vi "Branched Log Example.vi"() -> ()   [LabVIEW 2019]
doc: "This example shows logging data from multiple loops. At first, only one sink is active and then when another is added both loops will write to both logs (even though the wire is branched and isn't \"directly\" connected to the wire where the second sink is added.\n\nThis shows the DVR capability and the flexibility for event logs to be added on the fly."
uses:
  Log/Event Level.ctl
  Log/Log.lvclass/Log.ctl
  Layouts/JSONLayout/JSONLayout.lvclass
  C:/Development/Open Source/tsc-event-logger/Layouts/Layout.lvclass
  9e8dcfb1-bbfa-4add-8900-7eeb32d884c9.vi
  6aea5bb5-3dcc-47de-b7f9-df75227292dc.vi
  Log/Read Sinks.vi
  Log Sinks/Sink-Console/Sink-Console.lvclass
  C:/Development/Open Source/tsc-event-logger/Log Sinks/Log Sinks.lvclass
  Log Sinks/Sink-Console/Construct - Input.vi
  Log Sinks/Send Log Packet.vi
  Log/Log.lvclass
  TSC Event Logger.lvlib
panel:
  out "Closed?":bool
  in  "Arguments":string[](array[string])
  in  "Bottom Level":T1=enum."INFO"
  in  "Record Bottom Event":bool
  in  "Bottom Message":string="test"
  in  "Add JSON Console":bool
  out "Second Console":string
  out "First Console":string
  in  "Level":T1=enum."INFO"
  in  "Record Event":bool
  in  "Message":string="test"
  out "Error Out":errorcluster
  # "Run VI: both loops should be able to log to first console. \nThe second console is added with the add button in the top loop. \n-->Will the second console get the bottom loop messages after that?????"
  # "Top-Loop"
  # "Bottom-Loop"
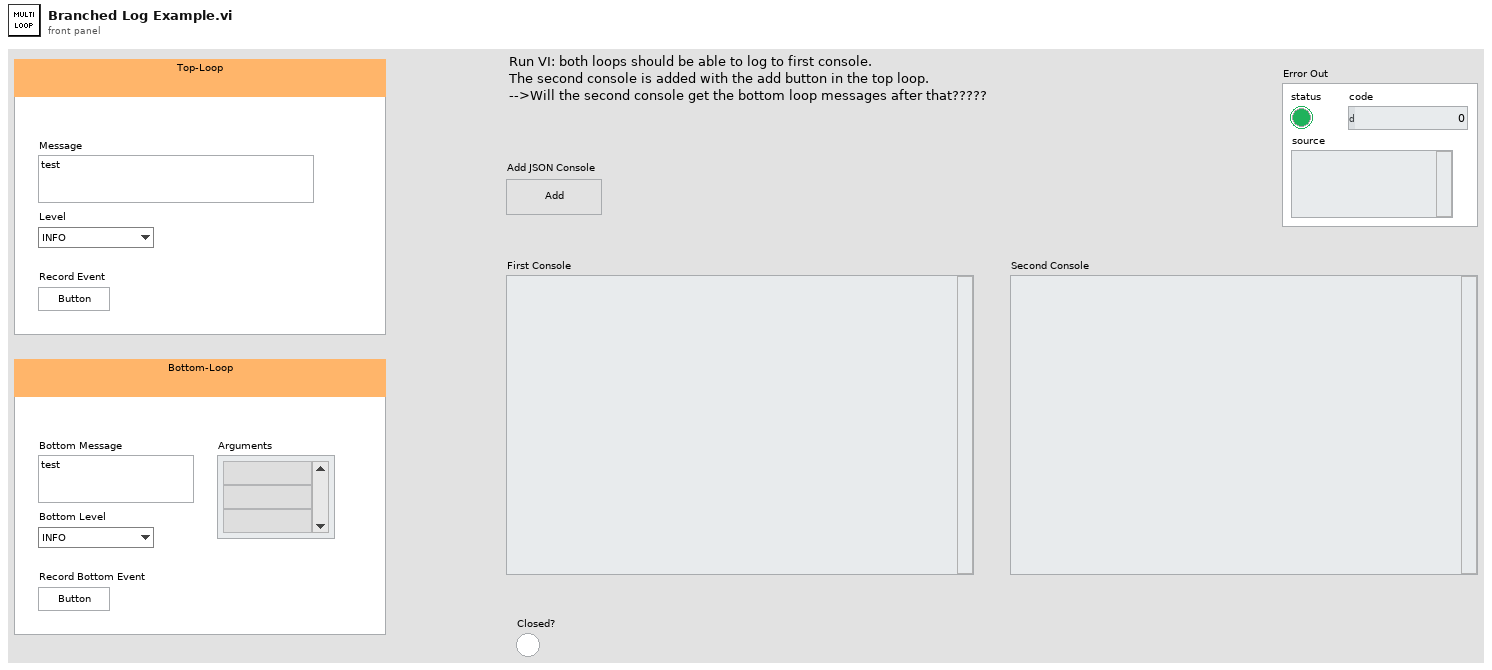
[diagram p1: front panel]
types:
  T1 = typedef "TSC Event Logger.lvlib/Event Level.ctl" = enum16{"OFF", "TRACE", "DEBUG", "INFO", "WARN", "ERROR", "FATAL"}
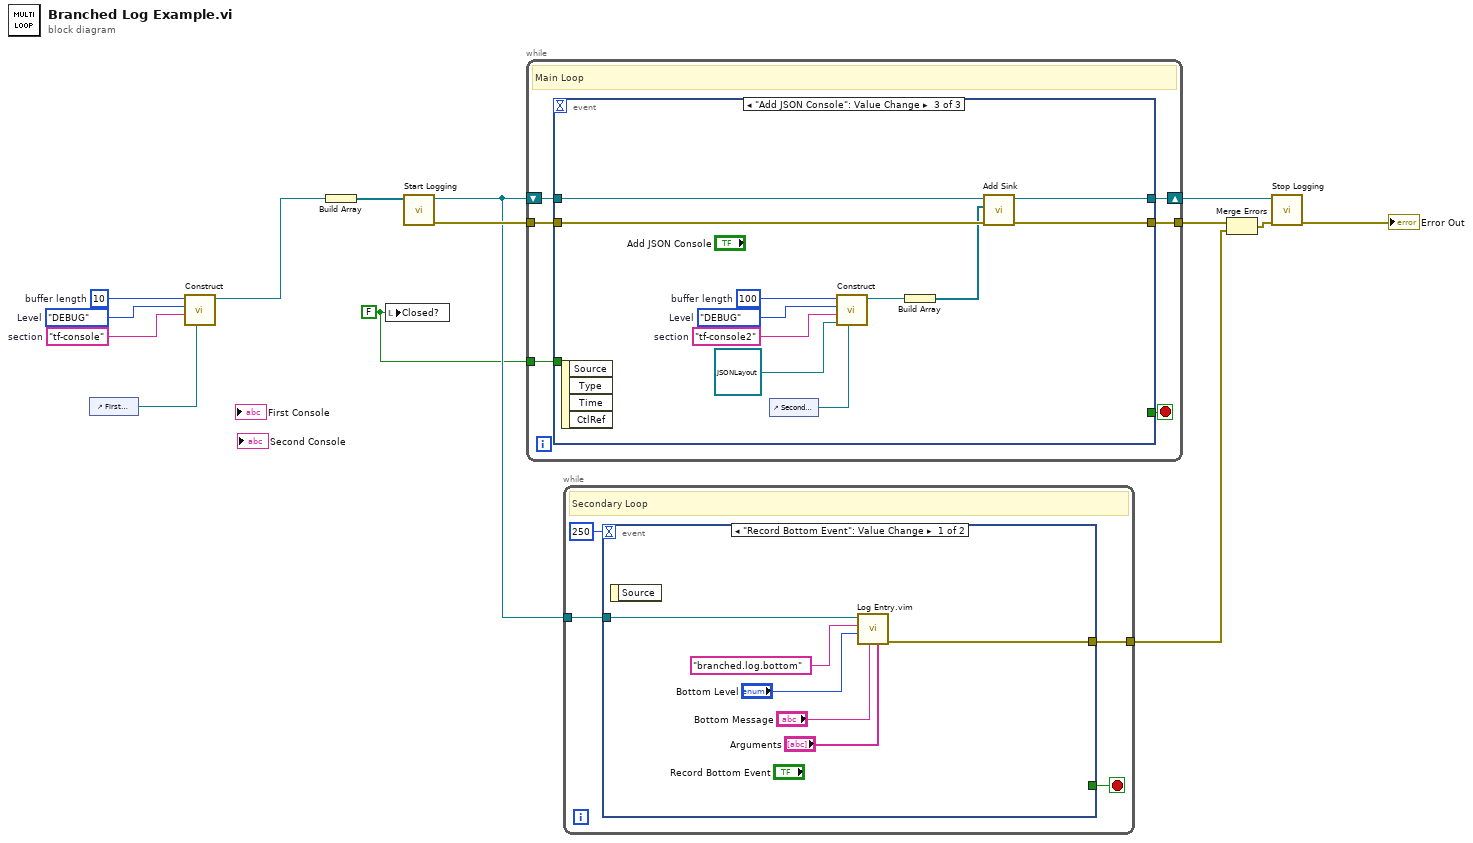
[diagram p0: block diagram]
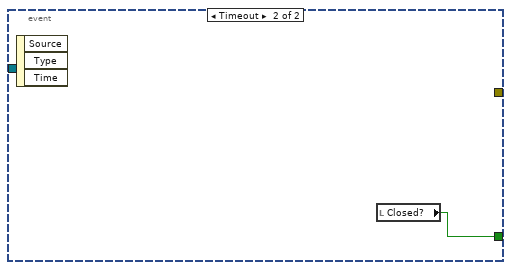
[diagram p2: hidden frame]
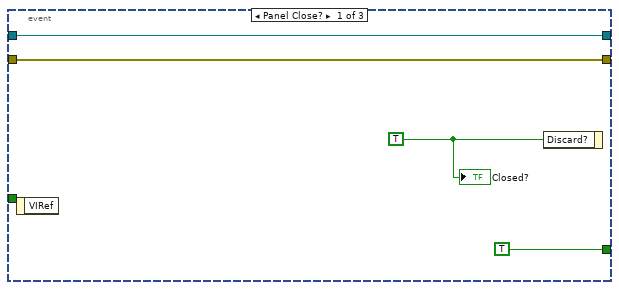
[diagram p3: hidden frame]
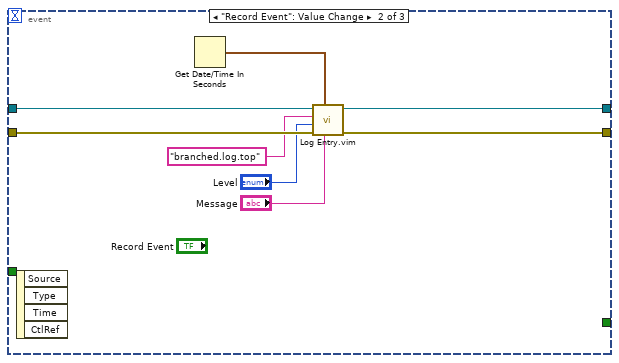
[diagram p4: hidden frame]
diagram:
  w1 = FALSE ("Closed?")
  w5 = 10  # buffer length
  w6 = Event_Level."DEBUG"  # Level
  w7 = "tf-console"  # section
  n1 = control-ref of="First Console"() -> (w8:refnum<vi>)
  n2 = call-poly "Construct.vi"("Console Ref"=w8, "Name"=w7, "Level"=w6, "buffer length"=w5) -> ("Sink-Console"=w9:refnum<class "Sink-Console.lvclass">)  [unwired: 6 in, 1 out]
  n3 = Build Array(w9) -> (w10:refnum<class "Sink-Console.lvclass">[])
  n4 = local write "Closed?"(w1) -> ()
  n5 = call "Start Logging.vi"("Sinks"=w10) -> ("Error Out"=w13:errorcluster, "Logger"=w4:refnum<class "Log.lvclass">)  [unwired: 9 in]
  n6 = while {
    tunnel: w13 -> [w19]
    shift-right: [w17] -> w12
    shift-left: w4 -> [w18]
    tunnel: [w16] -> w11
    tunnel: w1 -> [w15]
    stop <- w20 stop-if-true
    # "Main Loop"
    n7 = event shown="[2] \"Add JSON Console\": Value Change" {
      selector: _ -> [_ _ _]
      dyn-events: _ -> [_ _ _]
      timeout: _ -> [_ _ _]
      tunnel: [TRUE _ _] -> w20
      tunnel: w19 -> [w22 w30 w43]
      tunnel: w18 -> [w23 w32 w41]
      tunnel: [w23 w31 w40] -> w17
      tunnel: [w22 w29 w42] -> w16
      tunnel: w15 -> [_ _ _]
      event Panel Close? {
        w21 = TRUE ("Discard?")
        n8 = event-data() -> ()  [unwired: 1 in, 1 out]
        n9 = event-data("Discard?"=w21) -> ()  [unwired: 1 in, 1 out]
        "Closed?" <- w21
      }
      event "Record Event": Value Change {
        n10 = event-data() -> ()  [unwired: 1 in, 4 out]
        n11 = Get Date/Time In Seconds() -> (seconds since 1Jan1904=w27:timestamp)
        n12 = call "Log Entry.vim"("Message"="Message", "Time"=w27, "error in (no error)"=w30, "Level"="Level", "Logger"="branched.log.top", "Log in"=w32) -> ("error out"=w29:errorcluster, "Log out"=w31:refnum<class "Log.lvclass">)  [unwired: 4 in]
      }
      event "Add JSON Console": Value Change {
        w39 = 100  # buffer length
        w38 = Event_Level."DEBUG"  # Level
        w37 = "tf-console2"  # section
        n13 = event-data() -> ()  [unwired: 1 in, 4 out]
        n14 = control-ref of="Second Console"() -> (w36:refnum<vi>)
        n15 = call-poly "Construct.vi"("Console Ref"=w36, "Layout Type"=refnum<class "JSONLayout.lvclass"> refnum ("TSC Event Logger.lvlib:JSONLayout.lvclass"), "Name"=w37, "Level"=w38, "buffer length"=w39) -> ("Sink-Console"=w35:refnum<class "Sink-Console.lvclass">)  [unwired: 5 in, 1 out]
        n16 = Build Array(w35) -> (w34:refnum<class "Sink-Console.lvclass">[])
        n17 = call "Add Sink.vi"("Error In"=w43, "Sinks"=w34, "Logger in"=w41) -> ("Error Out"=w42:errorcluster, "Logger"=w40:refnum<class "Log.lvclass">)  [unwired: 7 in]
      }
    }
  }
  n18 = while {
    tunnel: w4 -> [w46]
    tunnel: [w45] -> w2
    stop <- w47 stop-if-true
    # "Secondary Loop"
    n19 = event shown="[0] \"Record Bottom Event\": Value Change" {
      selector: _ -> [_ _]
      dyn-events: _ -> [_ _]
      timeout: 250 -> [_ _]
      tunnel: [_ w54] -> w47
      tunnel: w46 -> [w52 _]
      tunnel: [w49 _] -> w45
      event "Record Bottom Event": Value Change {
        n20 = event-data() -> ()  [unwired: 1 in, 1 out]
        n21 = call "Log Entry.vim"("Arguments"="Arguments", "Message"="Bottom Message", "Level"="Bottom Level", "Logger"="branched.log.bottom", "Log in"=w52) -> ("error out"=w49:errorcluster)  [unwired: 5 in, 1 out]
      }
      event Timeout {
        n22 = event-data() -> ()  [unwired: 1 in, 3 out]
        n23 = local read "Closed?"() -> (w54:bool)
      }
    }
  }
  n24 = Merge Errors(w11, w2) -> (w3:errorcluster)
  n25 = call "Stop Logging.vi"("Error In"=w3, "Logger"=w12) -> ("Error Out"=→"Error Out":errorcluster)  [unwired: 8 in, 1 out]
